vi "From Veristand Master To Modbus.vi"(7 "Parameters":T1={"Interface Data"={"Name"="", "Unit ID"=0, "Refresh Rate"=0, "Write Rate"=0, "Write Mode"=enum."Value Change", "Interface Type"=enum."TCP Master", "TCP Settings"={"Address"="", "Port"=0, "Timeout"=0}, "Serial Settings"={"VISA resource name"="", "baud rate"=0, "parity (even)"=0, "flow control (none)"=0, "serial type"=enum."RTU", "Wire Mode"=-1}}, "Modbus Input Groups"=[], "Modbus Output Groups"=[], "error in (no error)"={"status"=FALSE, "code"=0, "source"=""}, "Modbus Input Engine Group Names"=[], "Modbus Output Engine Group Names"=[]} {"Modbus Output Groups"."Channel Data"."Mapping"."VS Reference" format="%.0x"; "Modbus Input Groups"."Channel Data"."Mapping"."VS Reference" format="%.0x"; "Interface Data"."Serial Settings"."Wire Mode" items=["Unknown"=-1, "RS485/Wire4"=0, "RS485/Wire2-EchoDTR"=1, "RS485/Wire2-CtrlDTR"=2, "RS485/Wire2-Auto"=3, "RS232/DTE"=128, "RS232/DCE"=129, "RS232/AUTO"=130]; "Interface Data"."Serial Settings"."parity (even)" items=["None", "Odd", "Even", "Mark", "Space"]; "Interface Data"."Serial Settings"."flow control (none)" items=["None", "XON/XOFF", "RTS/CTS", "XON/XOFF & RTS/CTS", "DTR/DSR", "XON/XOFF & DTR/DSR"]}, 8 "error in (no error)":errorcluster, 10 "Process in":refnum<class "Process.lvclass">, 11 "Modbus Master in":refnum<class "Modbus Master.lvclass">=refnum) -> ()   [LabVIEW 2021, in "Modbus Master Engine.lvlib"]
uses:
  Modbus Master Engine.lvlib
  <vilib>/NI/NIVS Inline Async API/_VS Inline Async API/Process/Process.lvclass
  Shared/Device Info.ctl
  Shared/Write Mode.ctl
  Shared/Controls/Interface Type.ctl
  Shared/Controls/Data Model/TCP Settings.ctl
  Shared/Controls/Data Model/Serial Settings.ctl
  Bulk Data Access.ctl
  System Explorer/SubVIs/Modbus Type.ctl
  Shared/Controls/Data Model/Channel.ctl
  <vilib>/NI VeriStand/Custom Device API/Custom Device Channel Type.ctl
  Shared/Controls/Data Model/Mapping.ctl
  Shared/Controls/Data Model/DataType.ctl
  <vilib>/NI VeriStand/Custom Device API/Custom Device Item Ref.ctl
  Modbus API.lvlibp/API/Master/Modbus Master.lvclass
  <vilib>/NI/NIVS Inline Async API/_Data Access Engine/Access Type Classes/Read/Read.lvclass/Read.ctl
  <vilib>/NI/NIVS Inline Async API/_VS Inline Async API/Process/Process.lvclass/Process.ctl
  <vilib>/NI/NIVS Inline Async API/_Data Access Engine/Data Access Engine/Methods/Read.Data.vi
  <vilib>/NI/NIVS Inline Async API/_VS Inline Async API/Error Handling Process/SubVIs/Error.ConvertArray.vi
  <vilib>/NI/NIVS Inline Async API/_Data Access Engine/Access Type Classes/Read/Read.ProcessData.vi
  <vilib>/NI/NIVS Inline Async API/_Data Access Engine/Data Access Engine/Data Access Engine.lvclass
  <vilib>/NI VeriStand/Custom Device Tools/Custom Device Utility Library/Custom Device Utility Library.lvlib
  <vilib>/NI/NIVS Inline Async API/_Data Access Engine/Access Type Classes/Write/Write.lvclass
  <vilib>/NI/NIVS Inline Async API/_Data Access Engine/Access Type Classes/Read/Read.lvclass
  Shared/Modbus Master Shared.lvlib
  <vilib>/NI VeriStand/Custom Device API/Custom Device API.lvlib
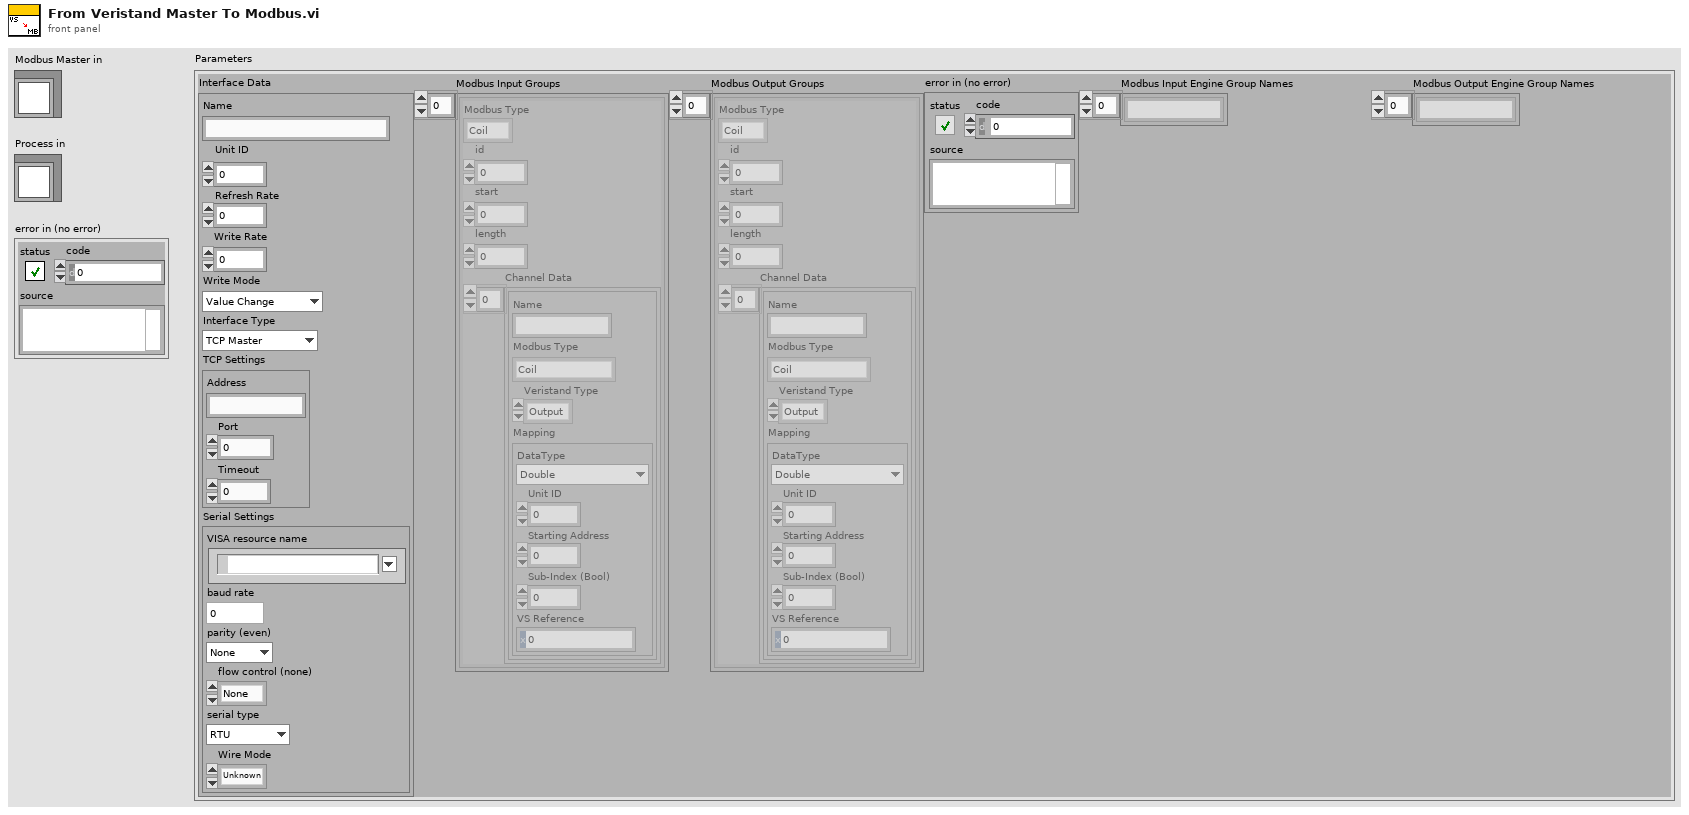
[diagram p1: front panel]
types:
  T1 = typedef "Modbus Master Shared.lvlib/Device Info.ctl" = cluster{"Interface Data":cluster{"Name":string, "Unit ID":u8, "Refresh Rate":i32, "Write Rate":i32, "Write Mode":T2, "Interface Type":T3, "TCP Settings":T4, "Serial Settings":T5}, "Modbus Input Groups":T6[], "Modbus Output Groups":T6[], "error in (no error)":errorcluster, "Modbus Input Engine Group Names":string[], "Modbus Output Engine Group Names":string[]}
  T2 = typedef "Modbus Master Shared.lvlib/Write Mode.ctl" = enum16{"Value Change", "Interval"}
  T3 = typedef "Modbus Master Shared.lvlib/Interface Type.ctl" = enum16{"TCP Master", "Serial Master", "TCP Slave", "Serial Slave"}
  T4 = typedef "Modbus Master Shared.lvlib/TCP Settings.ctl" = cluster{"Address":string, "Port":u16, "Timeout":i32}
  T5 = typedef "Modbus Master Shared.lvlib/Serial Settings.ctl" = cluster{"VISA resource name":refnum<visa-resource-name>, "baud rate":u32, "parity (even)":u16, "flow control (none)":u16, "serial type":enum16{"RTU", "ASCII"}, "Wire Mode":i16}
  T6 = typedef "Modbus Master Shared.lvlib/Bulk Data Access.ctl" = cluster{"Modbus Type":T7, "id":u8, "start":u16, "length":u16, "Channel Data":T8[]}
  T7 = typedef "Modbus Master Shared.lvlib/Modbus Type.ctl" = enum16{"Coil", "Discrete Input", "Holding Register", "Input Register"}
  T8 = typedef "Modbus Master Shared.lvlib/Channel.ctl" = cluster{"Name":string, "Modbus Type":T7, "Veristand Type":T9, "Mapping":T10}
  T9 = typedef "Custom Device API.lvlib/Custom Device Channel Type.ctl" = enum16{"Input", "Output"}
  T10 = typedef "Modbus Master Shared.lvlib/Mapping.ctl" = cluster{"DataType":T11, "Unit ID":u8, "Starting Address":u16, "Sub-Index (Bool)":u16, "VS Reference":T12}
  T11 = typedef "Modbus Master Shared.lvlib/DataType.ctl" = enum16{"Double", "Single", "I64", "I32", "I16", "I8", "U64", "U32", "U16", "U8", "Boolean"}
  T12 = typedef "Custom Device API.lvlib/Custom Device Item Ref.ctl" = u64
  T13 = typedef "Data Access Engine.lvlib/Data Access Engine.lvclass/Write.DVR.ctl" = refnum<data-value>
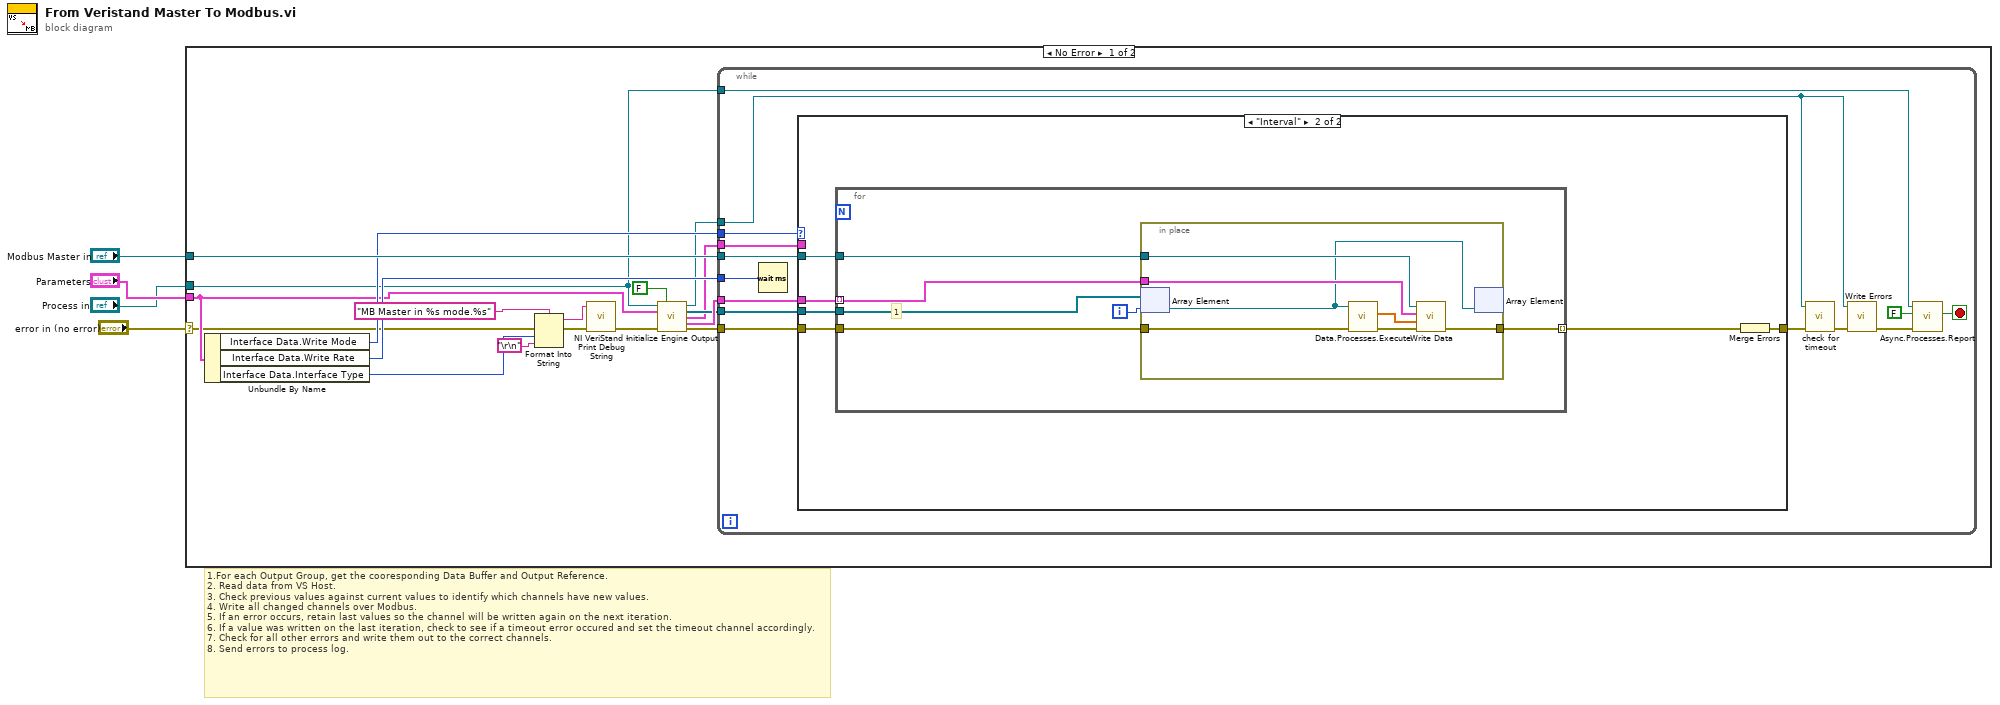
[diagram p0: block diagram]
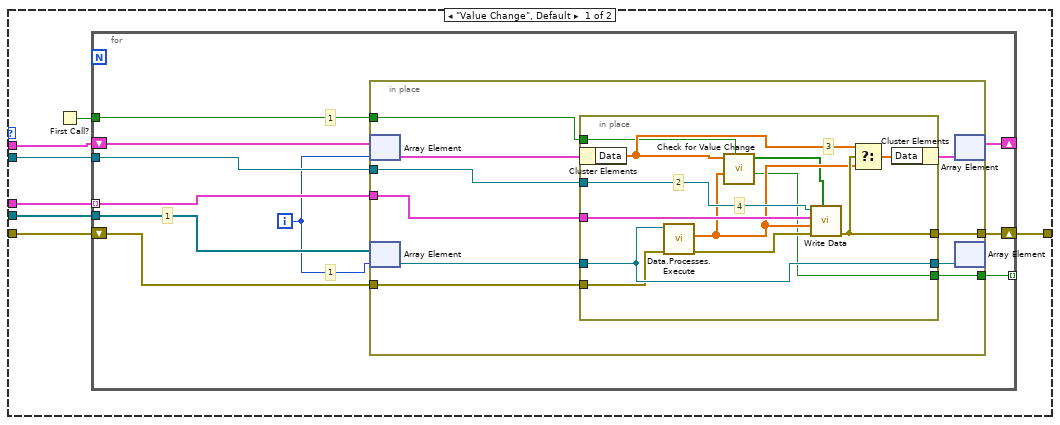
[diagram p2: hidden frame]
diagram:
  # "1.For each Output Group, get the cooresponding Data Buffer and Output Reference.\n2. Read data from VS Host.\n3. Check previous values against current values to identify which channels have new values.\n4. Write all changed channels over Modbus.\n5. If an error occurs, retain last values so the channel will be written again on the next iteration.\n6. If a value was written on the last iteration, check to see if a timeout error occured and set the timeout channel accordingly.\n7. Check for all other errors and write them out to the correct channels.\n8. Send errors to process log."
  n1 = case shown="No Error" "error in (no error)" {
    selector: "error in (no error)" -> [w5 _]
    tunnel: "Parameters" -> [w14 _]
    tunnel: "Modbus Master in" -> [w22 _]
    tunnel: "Process in" -> [w13 _]
    frame No Error {
      n2 = Unbundle By Name(w14) -> ("Interface Data.Write Mode"=w20:T2, "Interface Data.Write Rate"=w21:i32, "Interface Data.Interface Type"=w10:T3)
      n3 = Format Into String(format string="MB Master in %s mode.%s", error in=w5, w10, "\r\n") -> (resulting string=w18:string, error out=w12:errorcluster)  [unwired: 1 in]
      n4 = call <vilib>:"NI VeriStand - Print Debug String.vi"("error in (no error)"=w12, "Message"=w18) -> ("error out"=w19:errorcluster)  [unwired: 9 in]
      n5 = call "Initialize Engine Output.vi"("Process in"=w13, "Init Data Buffers? (T)"=FALSE, "Parameters"=w14, "error in (no error)"=w19) -> ("Diagnostic Group Ref"=w9:T13, "Output Group Refs"=w7:refnum<data-value>[], "Data Buffers"=w6:cluster{"Data":dbl[]}[], "Modbus Output Groups"=w8:T6[], "error out"=w11:errorcluster)  [unwired: 7 in]
      n6 = while {
        tunnel: w13 -> [w36]
        tunnel: w7 -> [w33]
        tunnel: w8 -> [w35]
        tunnel: w22 -> [w34]
        tunnel: w21 -> [w29]
        tunnel: w9 -> [w25]
        tunnel: w20 -> [w24]
        tunnel: w6 -> [w23]
        tunnel: w11 -> [w30]
        stop <- w32 stop-if-true
        n7 = Wait (ms)(milliseconds to wait=w29) -> ()  [unwired: 1 out]
        n8 = case shown="\"Interval\"" w24 {
          tunnel: w35 -> [w40 w81]
          tunnel: w34 -> [w41 w80]
          tunnel: w33 -> [w39 w79]
          tunnel: w30 -> [w38 w78]
          tunnel: [w37 w76] -> w27
          tunnel: w23 -> [w42 _]
          frame "Value Change", Default {
            n9 = First Call?() -> (First Call?: T/F=w43:bool)
            n10 = for {
              tunnel: w40 -> [w52] mode=indexing
              tunnel: w41 -> [w53]
              tunnel: w39 -> [w48]
              shift-right: [w49] -> _
              shift-left: w42 -> [w50]
              tunnel: w43 -> [w46]
              shift-right: [w45] -> w37
              shift-left: w38 -> [w51]
              tunnel: [w44] -> _ mode=indexing
              i -> [w47]
              # "1"
              # "1"
              # "1"
              n11 = in-place {
                in-place-border: w53 -> [w63]
                in-place-border: w52 -> [w62]
                in-place-border: w51 -> [w61]
                in-place-border: [w60] -> w45
                in-place-border: w46 -> [w55]
                in-place-border: [w54] -> w44
                n12 = in-place-array #1(w50, w47) -> (w59:cluster{"Data":dbl[]})
                n13 = in-place-array #2(w48, w47) -> (w57:refnum<data-value>)
                n14 = in-place {
                  in-place-border: w63 -> [w73]
                  in-place-border: w62 -> [w71]
                  in-place-border: w61 -> [w74]
                  in-place-border: [w70] -> w60
                  in-place-border: w57 -> [w75]
                  in-place-border: [w75] -> w56
                  in-place-border: w55 -> [w64]
                  in-place-border: [w66] -> w54
                  # "4"
                  # "3"
                  # "2"
                  n15 = in-place-cluster #3(w59) -> ("Data"=w68:dbl[])
                  n16 = call-poly <vilib>:"Data.Processes.Execute.vi"("error in (no error)"=w74, "Ref"=w75) -> ("error out"=w72:errorcluster, "Values"=w67:dbl[])  [unwired: 7 in, 1 out]
                  n17 = call "Check for Value Change.vi"("Force Write?"=w64, "New Data"=w67, "Last Value Data"=w68) -> ("Value Change?"=w66:bool, "Indices to Update"=w65:bool[])  [unwired: 7 in]
                  n18 = call "Write Data.vi"("Write Mask"=w65, "error in (no error)"=w72, "Values"=w67, "output data access"=w71, "Modbus Master in"=w73) -> ("error out"=w70:errorcluster)  [unwired: 6 in]
                  n19 = Select(t=w68, s=w70, f=w67) -> (s? t:f=w69:dbl[])
                  n20 = in-place-cluster #3("Data"=w69) -> (w58:cluster{"Data":dbl[]})
                }
                n21 = in-place-array #1(w58) -> (w49:cluster{"Data":dbl[]}[])  [unwired: 1 out]
                n22 = in-place-array #2(w56) -> ()  [unwired: 2 out]
              }
            }
          }
          frame "Interval" {
            n23 = for {
              tunnel: w81 -> [w86] mode=indexing
              tunnel: w80 -> [w87]
              tunnel: w79 -> [w84]
              tunnel: w78 -> [w85]
              tunnel: [w82] -> w77 mode=indexing
              i -> [w83]
              # "1"
              n24 = in-place {
                in-place-border: w87 -> [w94]
                in-place-border: w86 -> [w93]
                in-place-border: w85 -> [w92]
                in-place-border: [w91] -> w82
                n25 = in-place-array #4(w84, w83) -> (w90:refnum<data-value>)
                n26 = call-poly <vilib>:"Data.Processes.Execute.vi"("error in (no error)"=w92, "Ref"=w90) -> ("error out"=w89:errorcluster, "Values"=w88:dbl[])  [unwired: 7 in, 1 out]
                n27 = call "Write Data.vi"("error in (no error)"=w89, "Values"=w88, "output data access"=w93, "Modbus Master in"=w94) -> ("error out"=w91:errorcluster)  [unwired: 7 in]
                n28 = in-place-array #4(w90) -> ()  [unwired: 2 out]
              }
            }
            n29 = Merge Errors(w77) -> (w76:errorcluster)
          }
        }
        n30 = call "check for timeout.vi"("error in (no error)"=w27, "Data Value Reference in"=w25) -> ("error out"=w26:errorcluster)  [unwired: 9 in]
        n31 = call "Write Errors.vi"("error in (no error)"=w26, "Data Value Reference in"=w25) -> ("error out"=w28:errorcluster)  [unwired: 9 in]
        n32 = call <vilib>:"Async.Processes.Report.vi"("Error"=w28, "Stop Async on Error?"=FALSE ("Stop on Error?"), "Process in"=w36) -> ("Stop"=w32:bool)  [unwired: 7 in, 1 out]
      }
    }
    frame Error {
    }
  }
